vi "SOAP解析.vi"(7 "DATA":string, 8 "错误输入（无错误）":errorcluster, 10 "Headers":string[][](array[string])=[["Content-Type", "text/xml;charset=UTF-8"], ["SOAPAction", "\"http://tempuri.org/IUserRightVerifyServiceImpl/UserRightVerify\""], ["Connection", "Keep-Alive"], ["User-Agent", "Apache-HttpClient/4.1.1 (java 1.5)"]], 11 "URL":string) -> (0 "错误输出":errorcluster, 1 "headers":string caption="头部", 2 "body":string)   [LabVIEW 2015]
uses:
  <vilib>/httpClient/POSTBuffer.vi
  <vilib>/httpClient/LabVIEWHTTPClient.lvlib
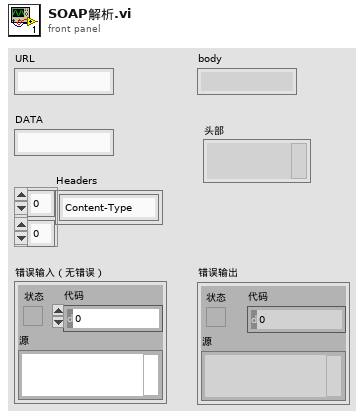
[diagram p1: front panel]
types:
  T1 = typedef "LabVIEWHTTPClient.lvlib/ClientHandle.ctl" = refnum<k1>
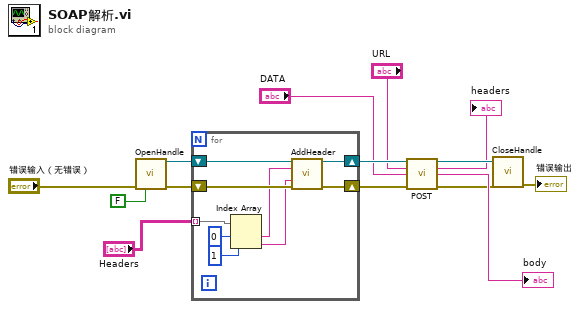
[diagram p0: block diagram]
diagram:
  n1 = call <vilib>:"OpenHandle.vi"("error in (no error)"="错误输入（无错误）", "verify server(true)"=FALSE) -> ("client handle out"=w11:T1, "error out"=w12:errorcluster)  [unwired: 12 in]
  n2 = for {
    shift-right: [w18] -> w10
    shift-left: w11 -> [w19]
    shift-right: [w20] -> w13
    shift-left: w12 -> [w21]
    tunnel: "Headers" -> [w15] mode=indexing
    n3 = Index Array(array=w15, index #1=0 ("index"), index #2=1 ("index")) -> (element #1=w17:string, element #2=w16:string)
    n4 = call <vilib>:"AddHeader.vi"("client handle"=w19, "header"=w17, "value"=w16, "error in (no error)"=w21) -> ("client handle out"=w18:T1, "error out"=w20:errorcluster)  [unwired: 10 in]
  }
  n5 = call-poly <vilib>:"POST.vi"("client handle"=w10, "url"="URL", "buffer"="DATA", "error in (no error)"=w13) -> ("client handle out"=w5:T1, "headers"=→"headers":string, "body"=→"body":string, "error out"=w4:errorcluster)  [unwired: 8 in]
  n6 = call <vilib>:"CloseHandle.vi"("client handle"=w5, "error in (no error)"=w4) -> ("error out"=→"错误输出":errorcluster)  [unwired: 13 in]
